vi "set window and buttons.vi"(0 "path in":path, 1 "expand ref":refnum<vi>, 5 "Shrink":bool, 7 "Window Dimensions":cluster{"width":i16, "height":i16}, 9 "Origin":T1, 11 "error in":errorcluster, 12 "shrink ref":refnum<vi>) -> (4 "path out":path, 15 "error out":errorcluster)   [LabVIEW 2016]
doc: "This subvi shrinks or expands the temp chart in the bottom right corner\n\nPaul K Dixon\nPhysics 350\nCSUSB Physics"
uses:
  <vilib>/Utility/miscctls.llb/LVPointTypeDef.ctl
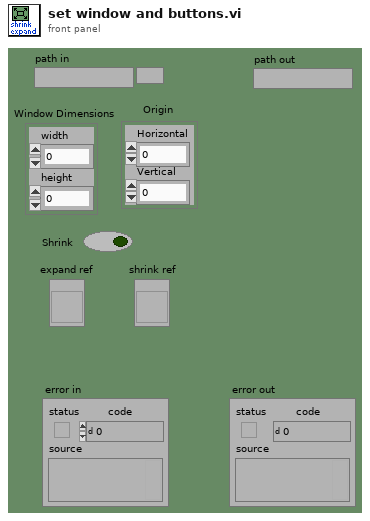
[diagram p1: front panel]
types:
  T1 = typedef "LVPointTypeDef.ctl" = cluster{"Horizontal":i16, "Vertical":i16}
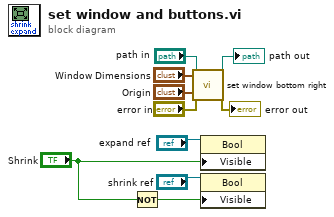
[diagram p0: block diagram]
diagram:
  n1 = Not(x="Shrink") -> (.not. x?=w4:bool)
  n2 = call "set window bottom right.vi"("path in"="path in", "Window Dimensions"="Window Dimensions", "Origin"="Origin", "error in (no error)"="error in") -> ("path out"=→"path out":path, "error out"=→"error out":errorcluster)  [unwired: 1 in, 9 out]
  n3 = property on="Property Node" class="Bool"(reference="expand ref", "Visible"="Shrink") -> ()  [unwired: 1 in, 2 out]
  n4 = property on="Property Node" class="Bool"(reference="shrink ref", "Visible"=w4) -> ()  [unwired: 1 in, 2 out]
